vi "LCV Actual Valve Position.vi"(8 "error in (no error)":errorcluster caption="Fehler (Eingang, kein Fehler)", 11 "Valve Handle":i64) -> (0 "error out":errorcluster caption="Fehler (Ausgang)", 3 "Actual valve position":i32)   [LabVIEW 2021, in "labbCAN_Valve_API.lvlib"]
doc: "LCV_Func long LCV_CALL LCV_ActualValvePosition(dev_hdl hValve);"
uses:
  labbCAN_Valve_API.lvlib
  labbCAN_Valve_API.dll
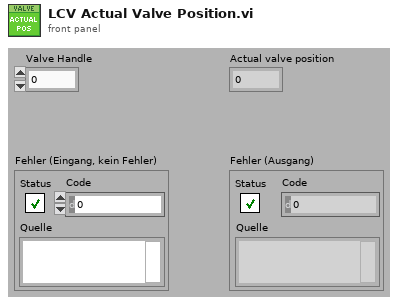
[diagram p1: front panel]
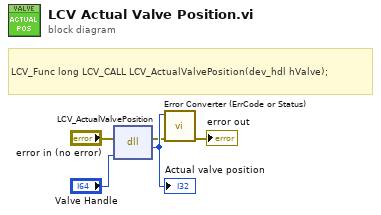
[diagram p0: block diagram]
diagram:
  # "LCV_Func long LCV_CALL LCV_ActualValvePosition(dev_hdl hValve);"
  n1 = dll-call lib="C:/Users/olaja/AppData/Local/CETONI_SDK/labbCAN_Valve_API.*" fn="LCV_ActualValvePosition"(error in="error in (no error)", "hValve"="Valve Handle") -> (error out=w2:errorcluster, "Rückgabetyp"=w5:i32)  [unwired: 3 in, 1 out]
  "Actual valve position" <- w5
  n2 = call "Error Converter (ErrCode or Status).vi"("error in (no error)"=w2, "error code"=w5) -> ("error out"=→"error out":errorcluster)  [unwired: 9 in]
